vi "DataType Cacher.vi"   [LabVIEW 2017]
doc: "Polymorphic wrapper that caches the description of a data type, so the same type is only analysed once."
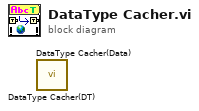
[diagram p0: block diagram]
diagram:
  n1 = call "DataType Cacher(DT).vi"() -> ()  [unwired: 8 in, 4 out]
  n2 = call "DataType Cacher(Data).vi"() -> ()  [unwired: 7 in, 5 out]
